vi "Get Spreadheet String.vi"(8 "error in (no error)":errorcluster, 10 "operation (0:open)":T1(ring), 11 "File Path":path) -> (0 "error out":errorcluster, 3 "Spreadsheet String":string)   [LabVIEW 2020]
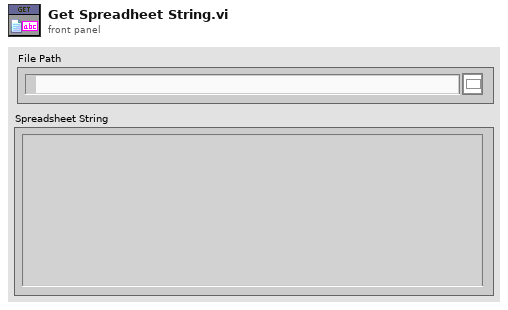
[diagram p1: front panel]
types:
  T1 = enum16{"open", "replace", "create", "open or create", "replace or create", "replace or create with confirmation"}
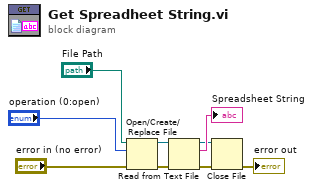
[diagram p0: block diagram]
diagram:
  n1 = Open/Create/Replace File(file path (use dialog)="File Path", error in="error in (no error)", operation (0:open)="operation (0:open)") -> (refnum out=w4:refnum<file>, error out=w3:errorcluster)  [unwired: 3 in, 1 out]
  n2 = Read from Text File(file (use dialog)=w4, error in=w3) -> (refnum out=w6:refnum<file>, text=→"Spreadsheet String":string, error out=w5:errorcluster)  [unwired: 2 in, 1 out]
  n3 = Close File(refnum=w6, error in=w5) -> (error out=→"error out":errorcluster)  [unwired: 1 out]
